vi "load_excel.vi"(11 "Path":path) -> (3 "data":string[][](array[string]))   [LabVIEW 2017]
uses:
  <vilib>/addons/_office/excel.llb/Excel Get Data ([str]).vi
  <vilib>/Utility/NIReport.llb/NI_report.lvclass
  <vilib>/Utility/NIReport.llb/Excel/NI_Excel.lvclass
  <vilib>/addons/_office/NI_ReportGenerationToolkit.lvlib
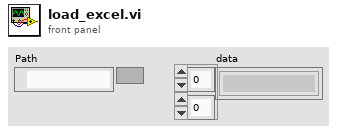
[diagram p1: front panel]
types:
  T1 = enum16{"Standard Report", "HTML", "Word", "Excel"}
  T2 = enum16{"maximized", "minimized", "normal", "no change"}
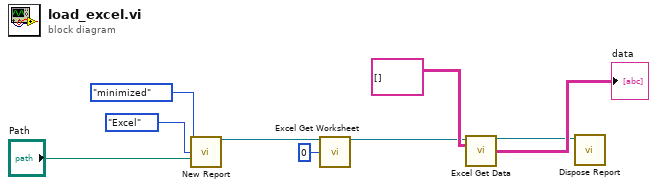
[diagram p0: block diagram]
diagram:
  n1 = call <vilib>:"New Report.vi"("window state (normal)"=T2."minimized", "report type"=T1."Excel", "template (empty)"="Path") -> ("report out"=w4:refnum<class "NI_report.lvclass">)  [unwired: 11 in, 1 out]
  n2 = call <vilib>:"Excel Get Worksheet.vi"("report in"=w4, "worksheet index (0)"=0) -> ("report out"=w6:refnum<class "NI_report.lvclass">)  [unwired: 12 in, 1 out]
  n3 = call-poly <vilib>:"Excel Get Data.vi"("report in"=w6, "data type"=string[][] [] ("Array")) -> ("report out"=w7:refnum<class "NI_report.lvclass">, "data"=→"data":string[][])  [unwired: 11 in, 1 out]
  n4 = call-dynamic "Dispose Report.vi"("report in"=w7) -> ()  [unwired: 14 in, 1 out]
